vi "WasInit.vi"(8 "No Error":errorcluster, 11 "Init Flags":T1 items=["NONE"=0, "SDL_INIT_AUDIO"=16, "SDL_INIT_VIDEO"=32, "SDL_INIT_JOYSTICK"=512, "SDL_INIT_HAPTIC"=4096, "SDL_INIT_GAMEPAD"=8192, "SDL_INIT_EVENTS"=16384, "SDL_INIT_SENSOR"=32768, "SDL_INIT_CAMER"=65536]) -> (0 "error out":errorcluster, 3 "Initialized Subsystems":T1 items=["NONE"=0, "SDL_INIT_AUDIO"=16, "SDL_INIT_VIDEO"=32, "SDL_INIT_JOYSTICK"=512, "SDL_INIT_HAPTIC"=4096, "SDL_INIT_GAMEPAD"=8192, "SDL_INIT_EVENTS"=16384, "SDL_INIT_SENSOR"=32768, "SDL_INIT_CAMER"=65536])   [LabVIEW 2026, in "SDL3.lvlib" / "Init.lvlib"]
doc: "<B>Summary</B>\nGet a mask of the specified subsystems which are currently initialized.\n\n<B>Remarks</B>\nReturns a mask of all initialized subsystems if flags is 0, otherwise it returns the initialization status of the specified subsystems."
uses:
  Init.lvlib
  InitFlags--ring.ctl
  Lib/SDL3.dll
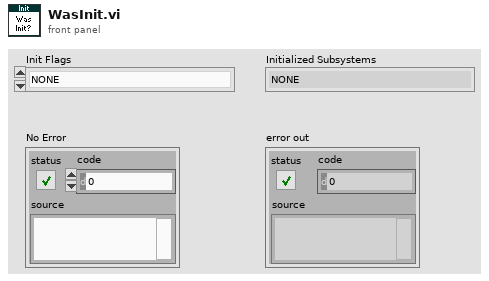
[diagram p1: front panel]
types:
  T1 = typedef "SDL3.lvlib/Init.lvlib/InitFlags--ring.ctl" = u32
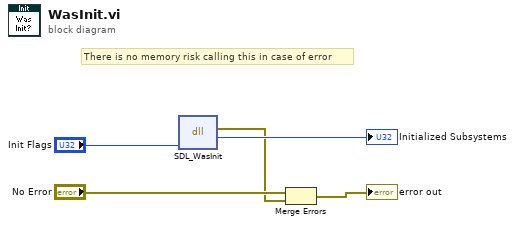
[diagram p0: block diagram]
diagram:
  # "There is no memory risk calling this in case of error"
  n1 = dll-call lib="C:/Users/saukko/Dev/LV-SDL3/Sources/SDL3/Lib/SDL3.*" fn="SDL_WasInit"("flags"="Init Flags") -> (error out=w1:errorcluster, "return type"=→"Initialized Subsystems":u32)  [unwired: 4 in, 1 out]
  n2 = Merge Errors("No Error", w1) -> (→"error out":errorcluster)
